vi "Matches.vi"(8 "error in (no error)":errorcluster, 10 "Actual":variant, 11 "IsTrue in":refnum<class "IsTrue.lvclass">) -> (0 "error out":errorcluster, 2 "Result":bool, 3 "IsTrue out":refnum<class "IsTrue.lvclass">)   [LabVIEW 2017, in "Transparent Assertions.lvlib" / "Constraints.lvlib" / "IsTrue.lvclass"]
doc: "Evaluates the constraint for <B>Actual</B>. Returns true if the constraint is met."
uses:
  IsTrue.lvclass
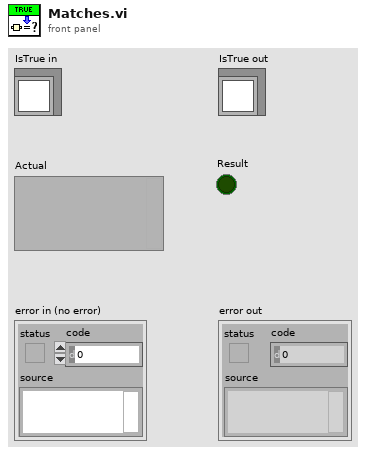
[diagram p1: front panel]
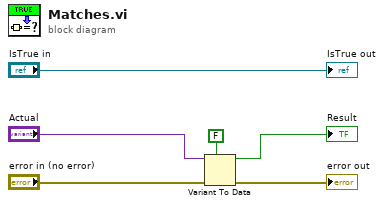
[diagram p0: block diagram]
diagram:
  n1 = Variant To Data(error in="error in (no error)", type=FALSE, Variant="Actual") -> (data=→"Result":bool, error out=→"error out":errorcluster)
  "IsTrue out" <- "IsTrue in"
